vi "FTW-BuildUtil-PreBuild Action.vi"(6 "Top Level/Always Included VIs":path[](array[path]), 7 "Main Destination Path":path, 9 "Target Name":string, 10 "Build Specification Name":string, 11 "Project Path":path) -> (0 "error out":errorcluster)   [LabVIEW 2013]
uses:
  <userlib>/_OpenG.lib/error/error.llb/Filter Error Codes (Array)__ogtk.vi
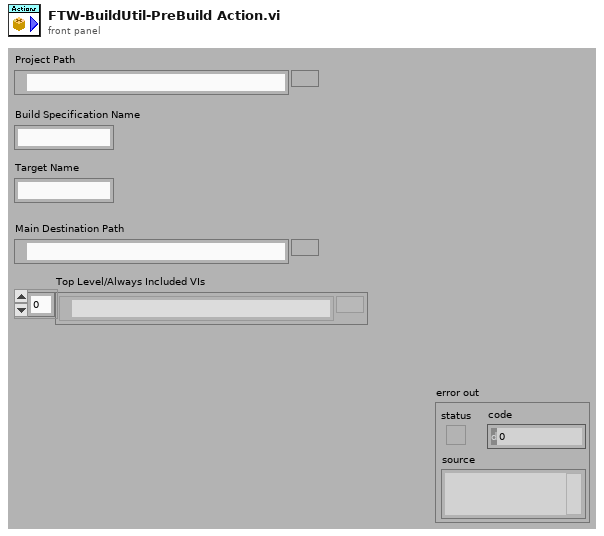
[diagram p1: front panel]
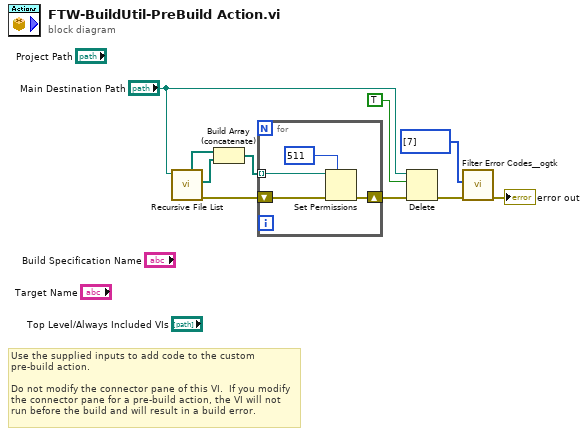
[diagram p0: block diagram]
diagram:
  # "Use the supplied inputs to add code to the custom pre-build action.\n\nDo not modify the connector pane of this VI.  If you modify the connector pane for a pre-build action, the VI will not run before the build and will result in a build error."
  n1 = call <vilib>:"Recursive File List.vi"("Folder Path"="Main Destination Path") -> ("error out"=w4:errorcluster, "All Files in Dir"=w1:path[], "All Folders"=w5:path[])  [unwired: 6 in, 2 out]
  n2 = Build Array (concatenate)(w5, w1) -> (w2:path[])
  n3 = for {
    tunnel: w2 -> [w14] mode=indexing
    shift-right: [w11] -> w3
    shift-left: w4 -> [w12]
    n4 = Set Permissions(7:i16 511 ("permissions"), 8:w12, 11:w14) -> (0:w11:errorcluster)  [unwired: 2 in, 1 out]
  }
  n5 = Delete(path (use dialog)="Main Destination Path", entire hierarchy (F)=TRUE, error in=w3) -> (error out=w9:errorcluster)  [unwired: 2 in, 2 out]
  n6 = call-poly <userlib>:"Filter Error Codes__ogtk.vi"("Error In"=w9, "Error Codes to Filter"=i32[] [7]) -> ("Error Out"=→"error out":errorcluster)  [unwired: 7 in, 2 out]
